vi "PDF Protokoll Linearisierung.vi"(8 "error in (no error)":errorcluster caption="Fehler (Eingang, kein Fehler)", 11 "Polynom-Ordnung":i32) -> (0 "error out":errorcluster caption="Fehler (Ausgang)")   [LabVIEW 2020, in "Linearisierung v2.lvlib" / "Protokoll.lvlib"]
uses:
  Protokoll.lvlib
  AktivArray.ctl
  AktivButton.ctl
  LIN Ausgabetabelle.ctl
  Polynomkoeffizientenanzeige.ctl
  Aktion Lin Daten aufarbeiten.ctl
  Seiten/FT-IR/FGV FT-IR Gasliste Aktionen.ctl
  <vilib>/Utility/miscctls.llb/LVPrintingMarginsTypeDef.ctl
  Linearisierung v2.lvlib
  Allgemein/allgemeine Sub-VIs.lvlib
  Seiten/FT-IR/FT-IR.lvlib
  Seiten/System Einstellungen V2/System Einstellungen V2.lvlib
panel:
  out "Gasflaschengenauigkeit":string caption="Genauigkeit:"
  out "Gasflaschennummer":string caption="Gasflasche:"
  out "Spanfaktor":string caption="Spanfaktor:"
  out "geforderte Genauigkeit":string caption="geforderte Genauigkeit:"
  out "Polynomkoeffizienten":T1 caption="Polynomkoeffizient:" {"O. 4" format="%#.10f"; "O. 3" format="%#.10f"; "O. 2" format="%#.10f"; "O.1" format="%#.10f"; "Offset" format="%#.10f"}
  out "Polynom-Ordnung":string caption="Polynom-Ordnung:"
  out "Ordnung festgelegt":string caption="Ordnung festgelegt:"
  out "erreichter max. Fehler (ppm)":string caption="erreichter max. Fehler (ppm):"
  out "erreichter max. Fehler (%)":string caption="erreichter max. Fehler (%):"
  out "geford. max. Fehler":string caption="geford. max. Fehler (% v. Sollw.):"
  out "LIN Ausgabetabelle":T2
  out "Aktiv":T3
  out "XY-Graph LIN":cluster{dbl[], dbl[]}[](graph) caption="XY-Graph"
  out "Datum:":string
  out "Konzentration:":string
  out "Komponente:":string
  out "Bearbeiter:":string
  out "Gasteiler:":string
  out "Messgerät:":string
  # "Linearity Check"
  # "Konstante"
  # "1.Ordnung"
  # "2.Ordnung"
  # "3.Ordnung"
  # "4.Ordnung"
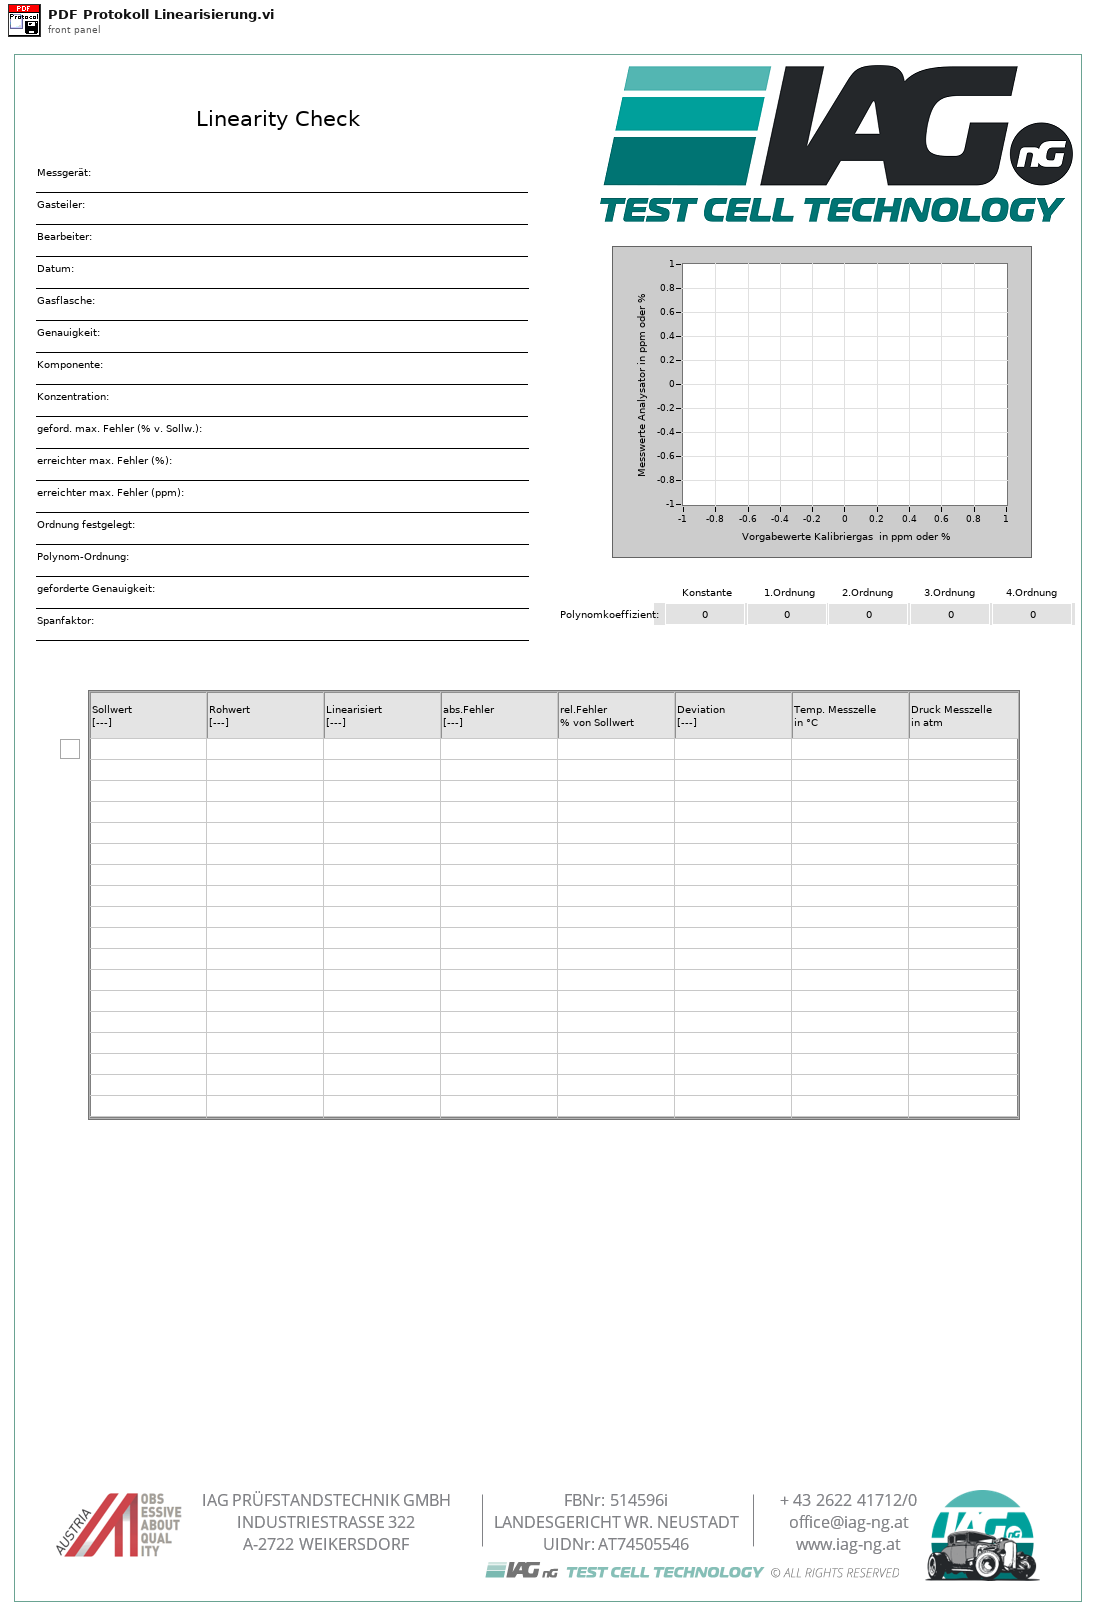
[diagram p1: front panel]
types:
  T1 = typedef "Linearisierung v2.lvlib/Polynomkoeffizientenanzeige.ctl" = cluster{"Offset":dbl, "O.1":dbl, "O. 2":dbl, "O. 3":dbl, "O. 4":dbl}
  T2 = typedef "Linearisierung v2.lvlib/LIN Ausgabetabelle.ctl" = string[][]
  T3 = typedef "Linearisierung v2.lvlib/AktivArray.ctl" = T4[]
  T4 = typedef "Linearisierung v2.lvlib/AktivButton.ctl" = bool
  T5 = typedef "FT-IR.lvlib/FGV FT-IR Gasliste Aktionen.ctl" = enum16{"lesen", "Gasliste FT-IR", "Gasliste ausgelesen", "laden", "speichern", "löschen"}
  T6 = typedef "Linearisierung v2.lvlib/Aktion Lin Daten aufarbeiten.ctl" = enum16{"lesen", "Protkolldaten", "speichern", "laden", "EPA auswerten", "Tabelle schreiben", "Lin auswerten", "Tab init", "Stufentabelle", "EPA aktiviert", "Nachbehandlung laden", "Tabelle löschen", "Istwerte löschen", "Zeile löschen", "Zeile einfügen", "LIN aktiviert", "LIN/EPA aktiv laden", "EGAK Tab", "LIN übernehmen", "Tab init ohne Stufen"}
  T7 = enum32{"Portrait", "Landscape", "Rotated Portrait", "Rotated Landscape"}
  T8 = typedef "LVPrintingMarginsTypeDef.ctl" = cluster{"Top":sgl, "Left":sgl, "Bottom":sgl, "Right":sgl, "Measurement System":enum8{"Inches", "cm"}}
  T9 = typedef "Auswahlfeld.ctl" = u16
  T10 = typedef "Linearisierung v2.lvlib/Eingabetabelle.ctl" = string[][]
  T11 = typedef "Linearisierung v2.lvlib/Lin-Polynom Daten.ctl" = cluster{"Messgerät":string, "Kalibrator (Gasteiler)":string, "Bearbeiter/in":string, "Komponente":string, "Zeitstempel":timestamp, "F_max gefordert (%)":sgl, "F_max in %":sgl, "F_max in ppm":sgl, "Vorschlag Ordnung":i32, "Polynom OK":bool, "Polynomkoeff.":dbl[], "Prüfgas Konzentration":dbl, "Pfad EPA":string, "Pfad_LIN":string, "Gasnummer:":u8, "Komponentenauswahl":T12, "Verdünnungsgas":T13, "Zeitdauer Stufe":T14, "Anzahl Stufen":T14, "F_max in % EPA":sgl, "F_max in ppm EPA":sgl, "F_max in % LIN":sgl, "F_max in ppm LIN":sgl, "Punkte umkehren":bool, "EPA Optionsfeld":T15, "Autolin Hovacal":T16, "Spanfactors":sgl[], "Kalibrierauswahl":T17, "Conditions:":T18, "Gasflaschen Nr.:":string, "Bottle Accuracy":dbl, "Konfig Gasflasche":T19, "Gasflasche":T20, "HovaCAL Flow AutoLin":T21, "MFC Output":T22, "Gas Ablaufdatum":timestamp, "Lin Modus":T23, "zusätzliche Zeitdauer Erster Punkt":sgl, "Offsets":sgl[]}
  T12 = typedef "Linearisierung v2.lvlib/KomponentenArray.ctl" = cluster{"Komponente:":T9, "Konzentration":dbl}[]
  T13 = typedef "Linearisierung v2.lvlib/Gasteiler.lvlib/Prüfgas in.ctl" = u16
  T14 = typedef "Zahlen-Eingabefeld.ctl" = sgl
  T15 = typedef "Linearisierung v2.lvlib/EPA Optionsfeld.ctl" = enum32{"Istwert", "Rohwert", "Linearisierter Wert"}
  T16 = typedef "Linearisierung v2.lvlib/Gasteiler.lvlib/HovaCal.lvlib/AutoLin Hovacal.ctl" = enum32{"Keine Auswahl", "Optionsauswahl 1", "Optionsauswahl 2"}
  T17 = typedef "Linearisierung v2.lvlib/Kalibrieroption.ctl" = u16
  T18 = typedef "Linearisierung v2.lvlib/Linearity verification 1065-307.lvlib/Condition.ctl" = u16
  T19 = typedef "System Einstellungen V2.lvlib/Konfig Gasflasche.ctl" = bool
  T20 = typedef "System Einstellungen V2.lvlib/Gasflasche Auswahl.ctl" = u16
  T21 = typedef "Linearisierung v2.lvlib/Gasteiler.lvlib/HovaCAL_Interface.lvlib/Controls.lvlib/Flow Einstellung.ctl" = cluster{"HovaCAL Flow Input Cluster":dbl}
  T22 = typedef "Linearisierung v2.lvlib/Gasteiler.lvlib/HovaCAL_Interface.lvlib/Controls.lvlib/Pump state.ctl" = cluster{"Run":bool}
  T23 = typedef "CalGas Aufschaltung.lvlib/Lin Modus.ctl" = u16
  T24 = cluster{"Polynomkoeff.[0]":dbl, "Polynomkoeff.[1]":dbl, "Polynomkoeff.[2]":dbl, "Polynomkoeff.[3]":dbl, "Polynomkoeff.[4]":dbl}
  T25 = typedef "String - Ausgabefeld.ctl" = string
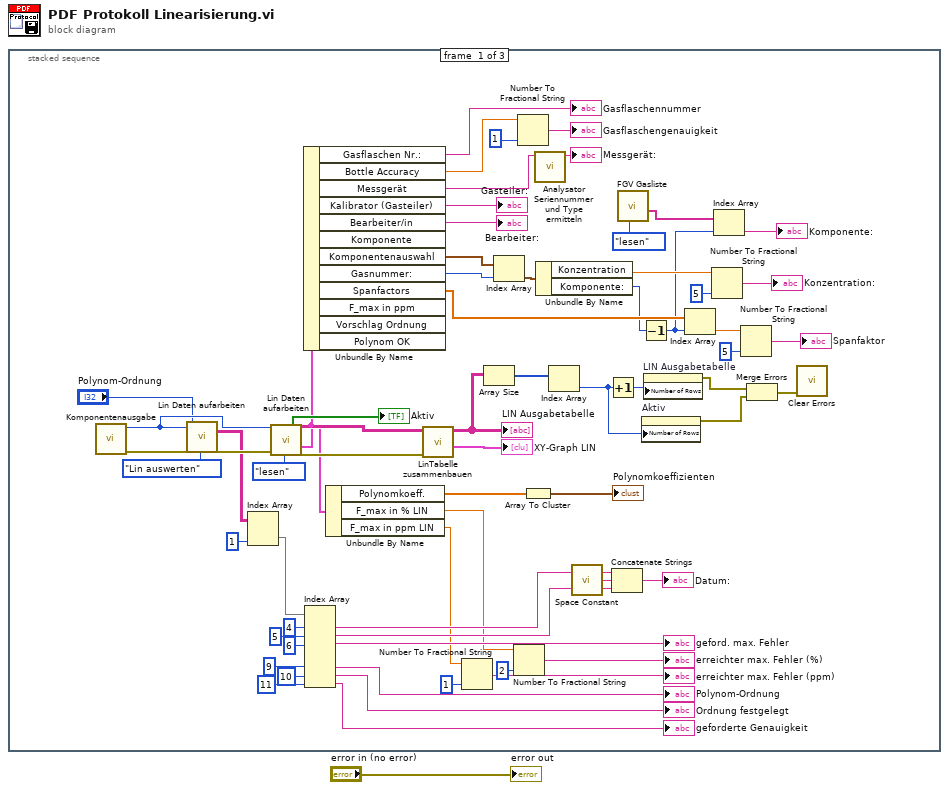
[diagram p0: block diagram]
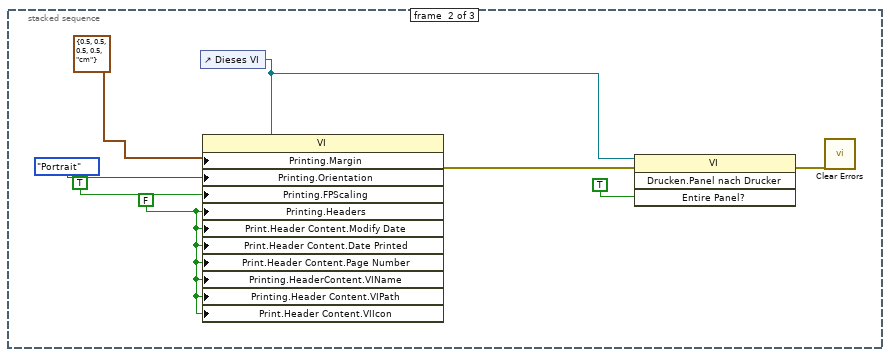
[diagram p2: hidden frame]
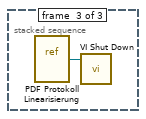
[diagram p3: hidden frame]
diagram:
  n1 = stacked-sequence {
    frame #0 {
      n2 = call "Komponentenausgabe.vi"() -> ("error out"=w58:errorcluster, "Gaskomponente"=w57:T9)  [unwired: 8 in, 2 out]
      n3 = call "Lin Daten aufarbeiten.vi"("Index (Seite)"=w57, "error in (no error)"=w58, "Polynom-Ordnung"="Polynom-Ordnung", "Aktionen"=Aktion_Lin_Daten_aufarbeiten."Lin auswerten") -> ("Ergebnis Lin"=w51:string[][], "error out"=w65:errorcluster)  [unwired: 13 in, 9 out]
      n4 = Index Array(array=w51, index (col)=1 ("Deaktivierter Index (Spalte)")) -> (element=w49:string[])  [unwired: 1 in]
      n5 = call "Lin Daten aufarbeiten.vi"("Index (Seite)"=w57, "error in (no error)"=w65, "Aktionen"=Aktion_Lin_Daten_aufarbeiten."lesen") -> ("Aktiv EPA"=→"Aktiv":T3, "Eingabetabelle"=w53:T10, "Lin-Polynom"=w34:T11, "error out"=w52:errorcluster)  [unwired: 14 in, 7 out]
      n6 = Unbundle By Name(w34) -> ("Gasflaschen Nr.:"=→"Gasflaschennummer":string, "Bottle Accuracy"=w6:dbl, "Messgerät"=w4:string, "Kalibrator (Gasteiler)"=→"Gasteiler:":string, "Bearbeiter/in"=→"Bearbeiter:":string, "Komponentenauswahl"=w63:T12, "Gasnummer:"=w62:u8, "Spanfactors"=w17:sgl[])  [unwired: 4 out]
      n7 = Index Array(array=w49, index #1=4 ("Index"), index #2=5 ("Index"), index #3=6 ("Index"), index #6=9 ("Index"), index #7=10 ("Index"), index #8=11 ("Index")) -> (element #1=w46:string, element #2=w44:string, element #3=→"geford. max. Fehler":string, element #6=→"Polynom-Ordnung":string, element #7=→"Ordnung festgelegt":string, element #8=→"geforderte Genauigkeit":string)  [unwired: 2 in, 2 out]
      n8 = Unbundle By Name(w34) -> ("Polynomkoeff."=w33:dbl[], "F_max in % LIN"=w23:sgl, "F_max in ppm LIN"=w21:sgl)
      n9 = call "LinTabelle zusammenbauen.vi"("error in (no error)"=w52, "Eingabetabelle"=w53) -> ("XY-Graph"=→"XY-Graph LIN":cluster{dbl[], dbl[]}[], "LIN Ausgabetabelle"=w31:string[][])  [unwired: 6 in, 2 out]
      "LIN Ausgabetabelle" <- w31
      n10 = Number To Fractional String(number=w21, precision (6)=i16 1 ("Genauigkeit (6)")) -> (F-format string=→"erreichter max. Fehler (ppm)":string)  [unwired: 2 in]
      n11 = Array Size(array=w31) -> (size(s)=w30:i32[])
      n12 = Index Array(array=w63, index=w62) -> (element=w61:cluster{"Komponente:":T9, "Konzentration":dbl})
      n13 = Number To Fractional String(number=w23, precision (6)=i16 2 ("Genauigkeit (6)")) -> (F-format string=→"erreichter max. Fehler (%)":string)  [unwired: 2 in]
      n14 = Number To Fractional String(number=w6, precision (6)=i16 1 ("Genauigkeit (6)")) -> (F-format string=→"Gasflaschengenauigkeit":string)  [unwired: 2 in]
      n15 = Array To Cluster(array=w33) -> (cluster=→"Polynomkoeffizienten":T24)
      n16 = call "Analysator Seriennummer und Type ermitteln.vi"("Analysator"=w4) -> ("Name für Protokoll"=→"Messgerät:":string)  [unwired: 8 in, 2 out]
      n17 = Unbundle By Name(w61) -> ("Konzentration"=w59:dbl, "Komponente:"=w16:T9)
      n18 = Index Array(array=w30) -> (element=w28:i32)  [unwired: 1 in]
      n19 = call <vilib>:"Space Constant.vi"() -> ("String"=w45:string)
      n20 = Increment(x=w28) -> (x+1=w29:i32)
      n21 = Concatenate Strings(w46, w45, w44) -> (→"Datum:":string)
      n22 = call "FGV Gasliste.vi"("Aktionen"=FGV_FT-IR_Gasliste_Aktionen."lesen") -> ("Aktuelle Gasliste gesamt"=w3:T25[])  [unwired: 8 in, 2 out]
      n23 = Decrement(x=w16) -> (x-1=w10:T9)
      n24 = property on="Aktiv" class="Arr"("Number of Rows"=w28) -> (error out=w26:errorcluster)  [unwired: 2 in, 1 out]
      n25 = property on="LIN Ausgabetabelle" class="Tbl (strikt)"("Number of Rows"=w29) -> (error out=w27:errorcluster)  [unwired: 2 in, 1 out]
      n26 = Index Array(array=w17, index=w10) -> (element=w13:sgl)
      n27 = Number To Fractional String(number=w59, precision (6)=i16 5 ("Genauigkeit (6)")) -> (F-format string=→"Konzentration:":string)  [unwired: 2 in]
      n28 = Index Array(array=w3, index=w10) -> (element=→"Komponente:":T25)
      n29 = Number To Fractional String(number=w13, precision (6)=i16 5 ("Genauigkeit (6)")) -> (F-format string=→"Spanfaktor":string)  [unwired: 2 in]
      n30 = Merge Errors(w27, w26) -> (w25:errorcluster)
      n31 = call <vilib>:"Clear Errors.vi"("error in (no error)"=w25) -> ()  [unwired: 5 in, 2 out]
    }
    frame #1 {
      w71 = FALSE ("Drucken:Kopfzeilen?")
      n32 = control-ref of="Dieses VI"() -> (w68:refnum<vi>)
      n33 = property class="VI"(reference=w68, "Printing.Margin"=T8 {"Top"=0.5, "Left"=0.5, "Bottom"=0.5, "Right"=0.5, "Measurement System"=enum."cm"} ("Drucken:Ränder"), "Printing.Orientation"=T7."Portrait" ("Drucken:Seitenausrichtung"), "Printing.FPScaling"=TRUE ("Drucken:Frontpanel-Skalierung?"), "Printing.Headers"=w71, "Print.Header Content.Modify Date"=w71, "Print.Header Content.Date Printed"=w71, "Print.Header Content.Page Number"=w71, "Printing.HeaderContent.VIName"=w71, "Printing.Header Content.VIPath"=w71, "Print.Header Content.VIIcon"=w71) -> (error out=w75:errorcluster)  [unwired: 1 in, 1 out]
      n34 = invoke class="VI" method="Drucken.Panel nach Drucker"(reference=w68, error in=w75, "Entire Panel?"=TRUE ("Abschnittskopfzeilen?")) -> (error out=w69:errorcluster)  [unwired: 1 in, 3 out]
      n35 = call <vilib>:"Clear Errors.vi"("error in (no error)"=w69) -> ()  [unwired: 5 in, 2 out]
    }
    frame #2 {
      n36 = vi-ref "PDF Protokoll Linearisierung.vi"() -> (w76:refnum<vi>)
      n37 = call "VI Shut Down.vi"("VI Referenz"=w76) -> ()  [unwired: 11 in]
    }
  }
  "error out" <- "error in (no error)"
